vi "BRig_RT_panel_ExpStruct_v1,10.vi"(7 "input_setValues":bool, 11 "input_dataExp":u16[](array[numeric])) -> (3 "output_dataExp":u16[](array[numeric]))   [LabVIEW 2014]
panel:
  in  "I_Cue2":bool
  in  "T_Cue2_LED_max":u16=1000 caption="Max" min=5 max=5000 step=5
  in  "T_Cue2_LED_min":u16=1000 caption="Min" min=5 max=5000 step=5
  in  "T_Cue2_LED_step":u16=1000 caption="Penalty" min=1 max=10000 step=1
  in  "T_Cue2_Audio_max":u16=1000 caption="Max" min=5 max=5000 step=5
  in  "T_Cue2_Audio_min":u16=1000 caption="Min" min=5 max=5000 step=5
  in  "T_Cue2_Audio_step":u16=1000 caption="Penalty" min=1 max=10000 step=1
  in  "T_ENL2_step":u16=100 caption="Penalty" min=10 max=10000 step=10
  in  "T_ENL2_max":u16=1000 caption="Max" min=250 max=10000 step=250
  in  "T_ENL2_min":u16=1000 caption="Min" min=250 max=10000 step=250
  in  "ClosedLoop_LaserHold_l2":bool
  in  "ClosedLoop_LaserHold_l1":bool
  in  "FreeReward_Count2":u16
  in  "FreeReward_Count1":u16
  in  "FreeReward_Switch":bool
  in  "T_CuePenalty":u16=1000 caption="Penalty" min=1 max=10000 step=1
  in  "T_ENLPenalty":u16=100 caption="Penalty" min=10 max=10000 step=10
  in  "LaserSwitch_Probability_L1":u16
  in  "LaserSwitch":u16(slide) max=3 step=1 scale=0.0..3.0
  in  "I_allReward":bool caption="NonSpecific Lick Direction"
  in  "Tcycle_Reward_max_R":u16=1000 caption="Max" min=5 max=5000 step=5
  in  "Tcycle_Reward_min_R":u16=1000 caption="Min" min=5 max=5000 step=5
  in  "Tcycle_Reward_step_R":u16=1000 caption="Penalty" min=1 max=10000 step=1
  in  "Tcycle_Reward_max_L":u16=1000 caption="Max" min=5 max=5000 step=5
  in  "Tcycle_Reward_min_L":u16=1000 caption="Min" min=5 max=5000 step=5
  in  "Tcycle_Reward_step_L":u16=1000 caption="Penalty" min=1 max=10000 step=1
  in  "T_Cue_LED_max":u16=1000 caption="Max" min=5 max=5000 step=5
  in  "T_Cue_LED_min":u16=1000 caption="Min" min=5 max=5000 step=5
  in  "T_Cue_LED_step":u16=1000 caption="Penalty" min=1 max=10000 step=1
  in  "SolenoidProbability_L":u16=100 caption="Reward Time [ms]" min=1 max=1000 step=1
  in  "SolenoidProbability_R":u16=100 caption="Reward Time [ms]" min=1 max=1000 step=1
  in  "T_Cue_Audio_max":u16=1000 caption="Max" min=5 max=5000 step=5
  in  "T_Cue_Audio_min":u16=1000 caption="Min" min=5 max=5000 step=5
  in  "BUR_max":u16 caption="Count Reward Structure  (0 = off)"
  in  "Tcycle_Timeout":u16=1000 caption="Timeout Time [ms]" min=10 max=10000 step=1
  in  "Tcycle_Wrong":u16=1000 caption="Wrong Time [ms]" min=10 max=10000 step=1
  in  "Tcycle_Selection":u16=1000 caption="Answer Time [ms]" min=1 max=10000 step=1
  in  "Tcycle_RewardPost":u16=1000 caption="Consumption Time [ms]" min=250 max=10000 step=250
  in  "TpB_Max_R":u16=4 caption="Max TrialsPerBlock" min=1 max=12 step=1
  in  "TpB_Min_R":u16=4 caption="Min TrialsPerBlock" min=1 max=12 step=1
  in  "TpB_Max_L":u16=4 caption="Max TrialsPerBlock" min=1 max=12 step=1
  in  "TpB_Min_L":u16=4 caption="Min TrialsPerBlock" min=1 max=12 step=1
  in  "BUR_min":u16 caption="Count Reward Structure\n(0 = off)"
  in  "TrialUntilReward":bool caption="Ignore Wrong Selection"
  in  "T_Cue_Audio_step":u16=1000 caption="Penalty" min=1 max=10000 step=1
  in  "T_ENL_step":u16=100 caption="Penalty" min=10 max=10000 step=10
  in  "T_ENL_max":u16=1000 caption="Max" min=250 max=10000 step=250
  in  "T_ENL_min":u16=1000 caption="Min" min=250 max=10000 step=250
  # "Experiment Task Structure"
  # "Min            Max               Step        Penalty"
  # "(Laser1 or Laser2)\nLaser1 probability"
  # "Enforced\nNonLick"
  # "Cue Audio"
  # "(ClosedLoop Structure)"
  # "Hold Laser1"
  # "Hold Laser2"
  # "Cue LED"
  # "Min            Max               Step"
  # "ENL 2"
  # "Cue 2 Audio"
  # "Cue 2 LED"
  # "Selection"
  # "Min"
  # "Max"
  # "Reward - Dispense Water"
  # "Min            Max            StepSize"
  # "Left"
  # "Trial Per Block Structure \n               Left                        Right"
  # "Right"
  # "Min"
  # "Dispense Water Probability"
  # "Max"
  # "%"
  # "Left"
  # "Right"
  # "%"
  # "Give Reward\nIf Too Many Errors"
  # "Reward - Consumption"
  # "# consecutive ReBiasing trials"
  # "Penalty - Wrong Choice"
  # "# consecutive NonForcedError trials"
  # "Penalty - Choice Timeout"
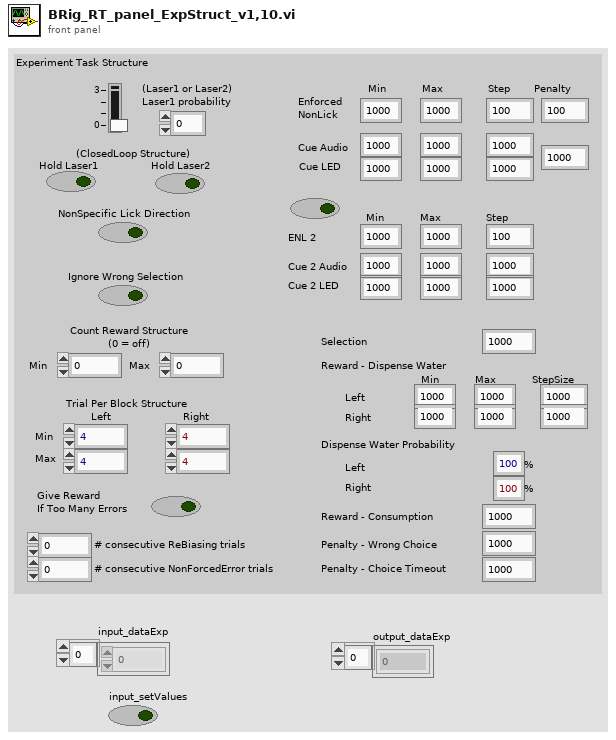
[diagram p1: front panel]
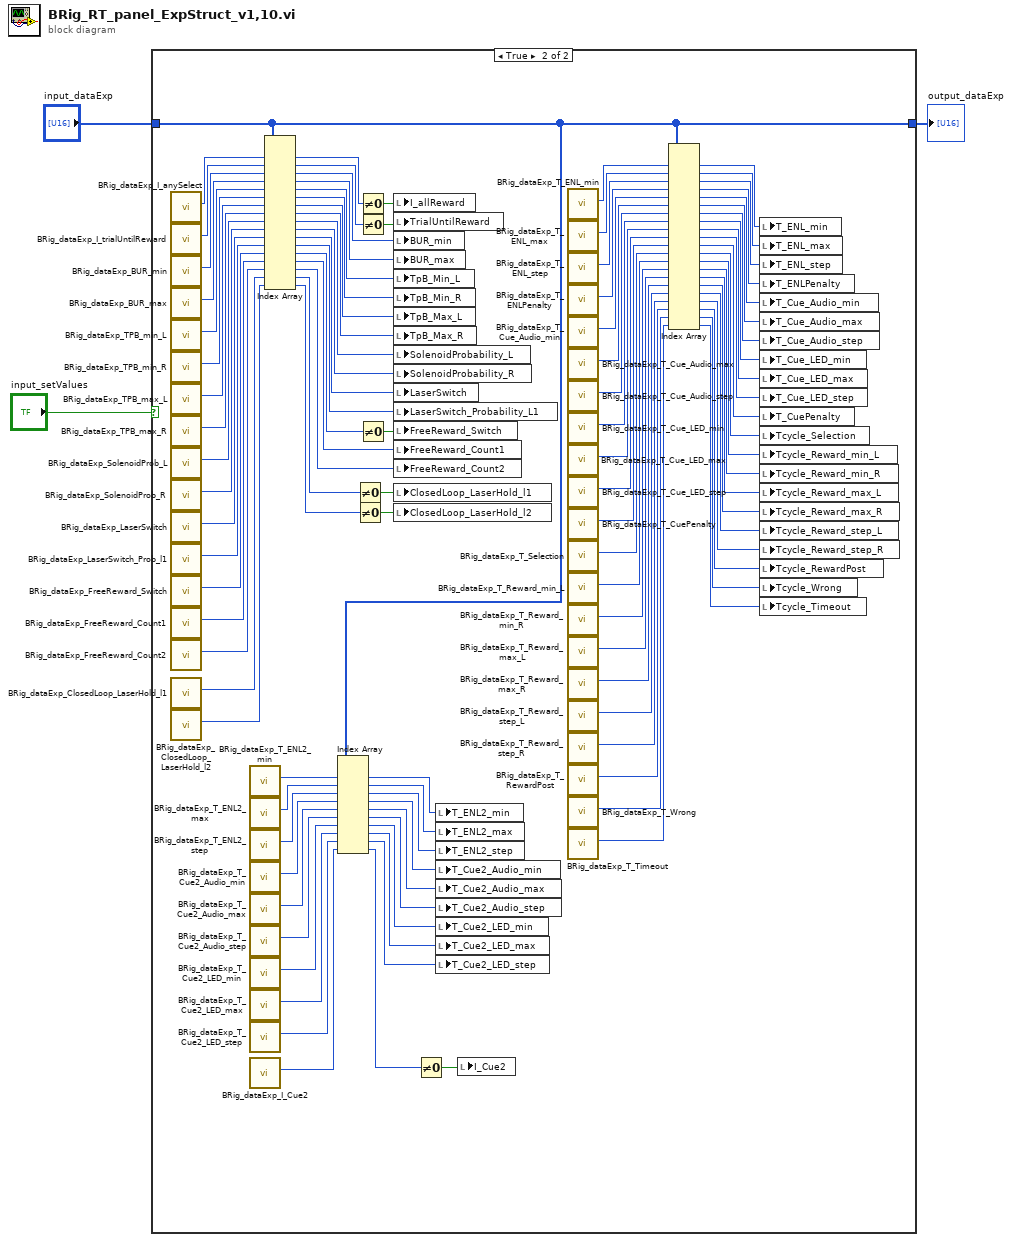
[diagram p0: block diagram]
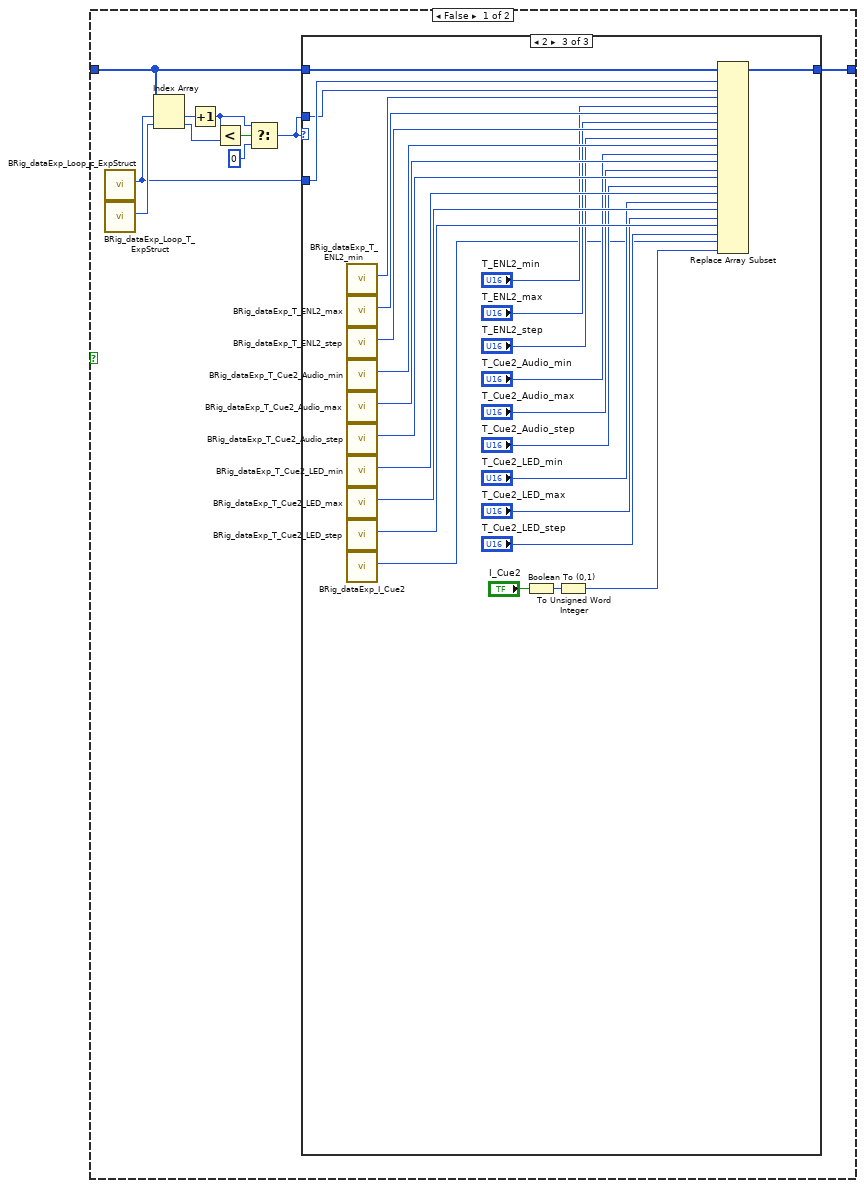
[diagram p2: hidden frame]
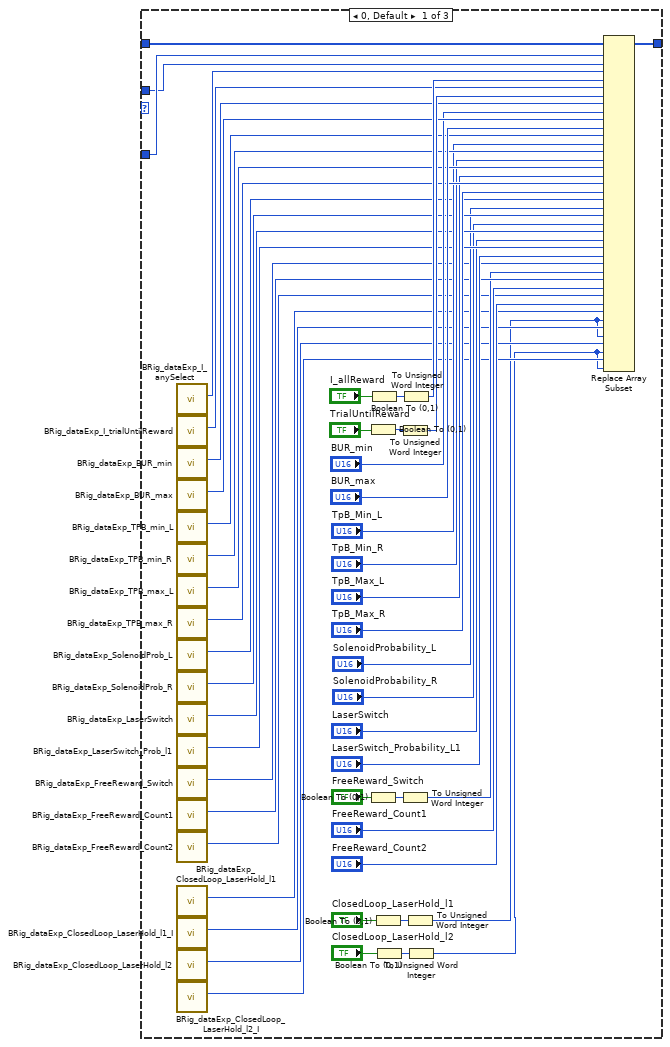
[diagram p3: hidden frame]
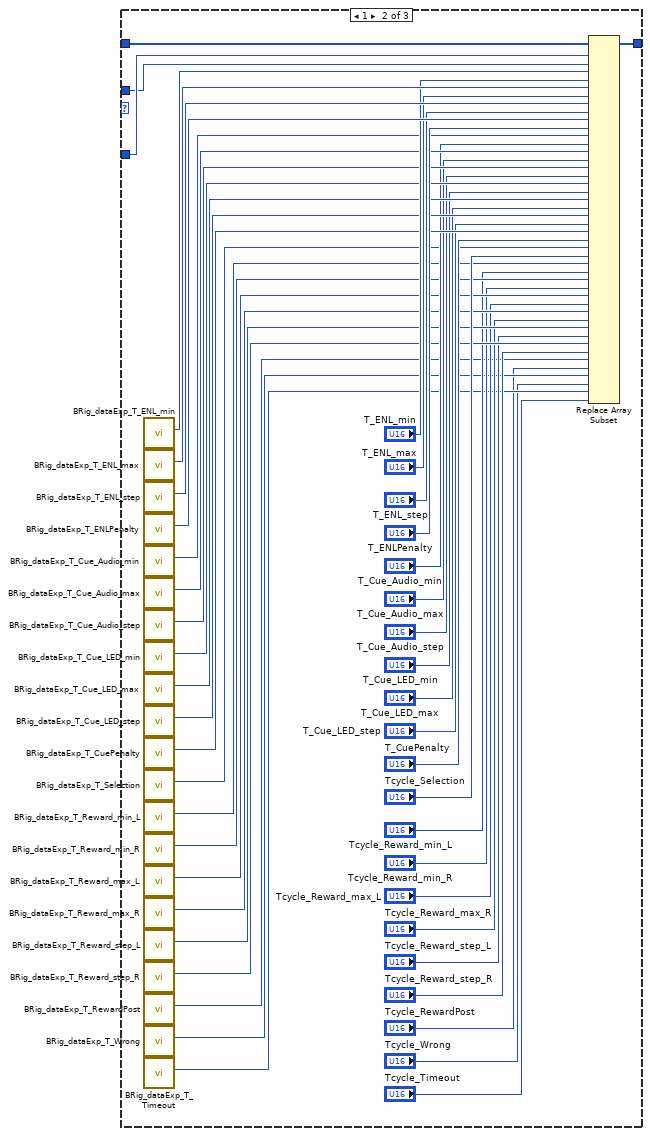
[diagram p4: hidden frame]
diagram:
  n1 = case shown="True" "input_setValues" {
    tunnel: [w13 w157] -> w3
    tunnel: "input_dataExp" -> [w12 w157]
    frame False {
      n2 = call "BRig_dataExp_Loop_c_ExpStruct.vi"() -> ("output_Loop_c_ExpStruct"=w6:i32)  [unwired: 11 in]
      n3 = call "BRig_dataExp_Loop_T_ExpStruct.vi"() -> ("output_Loop_T_ExpStruct"=w11:i32)  [unwired: 11 in]
      n4 = Index Array(array=w12, index #1=w6, index #2=w11) -> (element #1=w10:u16, element #2=w9:u16)
      n5 = Increment(x=w10) -> (x+1=w5:u16)
      n6 = Less?(x=w5, y=w9) -> (x < y?=w8:bool)
      n7 = Select(t=w5, s=w8, f=u16 0) -> (s? t:f=w4:u16)
      n8 = case shown="2" w4 {
        tunnel: w12 -> [w63 w109 w135]
        tunnel: [w62 w108 w134] -> w13
        tunnel: w6 -> [w33 w107 w133]
        tunnel: w4 -> [w32 w106 w132]
        frame 0, Default {
          n9 = call "BRig_dataExp_I_anySelect.vi"() -> ("output_I_anySelect"=w61:i32)  [unwired: 11 in]
          n10 = call "BRig_dataExp_I_trialUntilReward.vi"() -> ("output_I_trialUntilReward"=w57:i32)  [unwired: 11 in]
          n11 = call "BRig_dataExp_BUR_min.vi"() -> ("output_BUR_min"=w53:i32)  [unwired: 11 in]
          n12 = call "BRig_dataExp_BUR_max.vi"() -> ("output_BUR_max"=w52:i32)  [unwired: 11 in]
          n13 = call "BRig_dataExp_TPB_min_L.vi"() -> ("output_TPB_min_L"=w49:i32)  [unwired: 11 in]
          n14 = call "BRig_dataExp_TPB_min_R.vi"() -> ("output_TPB_min_R"=w48:i32)  [unwired: 11 in]
          n15 = call "BRig_dataExp_TPB_max_L.vi"() -> ("output_TPB_max_L"=w47:i32)  [unwired: 11 in]
          n16 = call "BRig_dataExp_TPB_max_R.vi"() -> ("output_TPB_max_R"=w46:i32)  [unwired: 11 in]
          n17 = call "BRig_dataExp_SolenoidProb_L.vi"() -> ("output_SolenoidProbability_L"=w41:i32)  [unwired: 11 in]
          n18 = call "BRig_dataExp_SolenoidProb_R.vi"() -> ("output_SolenoidProbability_R"=w40:i32)  [unwired: 11 in]
          n19 = call "BRig_dataExp_LaserSwitch.vi"() -> ("output_LaserSwitch"=w39:i32)  [unwired: 11 in]
          n20 = call "BRig_dataExp_LaserSwitch_Prob_l1.vi"() -> ("output_LaserSwitch_Probability_L1"=w38:i32)  [unwired: 11 in]
          n21 = call "BRig_dataExp_FreeReward_Switch.vi"() -> ("output_FreeReward_Switch"=w29:i32)  [unwired: 11 in]
          n22 = call "BRig_dataExp_FreeReward_Count1.vi"() -> ("output_FreeReward_Count"=w28:i32)  [unwired: 11 in]
          n23 = call "BRig_dataExp_FreeReward_Count2.vi"() -> ("output_FreeReward_Count"=w25:i32)  [unwired: 11 in]
          n24 = call "BRig_dataExp_ClosedLoop_LaserHold_l1.vi"() -> ("output_CloseLoop_LaserHold_l1"=w23:i32)  [unwired: 11 in]
          n25 = call "BRig_dataExp_ClosedLoop_LaserHold_l1_I.vi"() -> ("output_CloseLoop_LaserHold_l1_I"=w22:i32)  [unwired: 11 in]
          n26 = call "BRig_dataExp_ClosedLoop_LaserHold_l2.vi"() -> ("output_CloseLoop_LaserHold_l2"=w21:i32)  [unwired: 11 in]
          n27 = call "BRig_dataExp_ClosedLoop_LaserHold_l2_I.vi"() -> ("output_CloseLoop_LaserHold_l2_I"=w20:i32)  [unwired: 11 in]
          n28 = Boolean To (0,1)(Boolean="TrialUntilReward") -> (0, 1=w56:i16)
          n29 = Boolean To (0,1)(Boolean="FreeReward_Switch") -> (0, 1=w31:i16)
          n30 = Boolean To (0,1)(Boolean="I_allReward") -> (0, 1=w59:i16)
          n31 = Boolean To (0,1)(Boolean="ClosedLoop_LaserHold_l1") -> (0, 1=w19:i16)
          n32 = Boolean To (0,1)(Boolean="ClosedLoop_LaserHold_l2") -> (0, 1=w17:i16)
          n33 = To Unsigned Word Integer(number=w56) -> (unsigned 16bit integer=w54:u16)
          n34 = To Unsigned Word Integer(number=w31) -> (unsigned 16bit integer=w27:u16)
          n35 = To Unsigned Word Integer(number=w59) -> (unsigned 16bit integer=w58:u16)
          n36 = To Unsigned Word Integer(number=w19) -> (unsigned 16bit integer=w15:u16)
          n37 = To Unsigned Word Integer(number=w17) -> (unsigned 16bit integer=w14:u16)
          n38 = Replace Array Subset(array=w63, new element #1=w32, index #1=w33, new element #2=w58, index #2=w61, new element #3=w54, index #3=w57, new element #4="BUR_min", index #4=w53, new element #5="BUR_max", index #5=w52, new element #6="TpB_Min_L", index #6=w49, new element #7="TpB_Min_R", index #7=w48, new element #8="TpB_Max_L", index #8=w47, new element #9="TpB_Max_R", index #9=w46, new element #10="SolenoidProbability_L", index #10=w41, new element #11="SolenoidProbability_R", index #11=w40, new element #12="LaserSwitch", index #12=w39, new element #13="LaserSwitch_Probability_L1", index #13=w38, new element #14=w27, index #14=w29, new element #15="FreeReward_Count1", index #15=w28, new element #16="FreeReward_Count2", index #16=w25, new element #17=w15, index #17=w23, new element #18=w15, index #18=w22, new element #19=w14, index #19=w21, new element #20=w14, index #20=w20) -> (w62:u16[])
        }
        frame 1 {
          n39 = call "BRig_dataExp_T_ENL_min.vi"() -> ("output_T_ENL_min"=w105:i32)  [unwired: 11 in]
          n40 = call "BRig_dataExp_T_ENL_max.vi"() -> ("output_T_ENL_max"=w104:i32)  [unwired: 11 in]
          n41 = call "BRig_dataExp_T_ENL_step.vi"() -> ("output_T_ENL_step"=w103:i32)  [unwired: 11 in]
          n42 = call "BRig_dataExp_T_ENLPenalty.vi"() -> ("output_ENL_penalty"=w102:i32)  [unwired: 11 in]
          n43 = call "BRig_dataExp_T_Cue_Audio_min.vi"() -> ("output_T_Cue_Audio_min"=w97:i32)  [unwired: 11 in]
          n44 = call "BRig_dataExp_T_Cue_Audio_max.vi"() -> ("output_T_Cue_Audio_max"=w96:i32)  [unwired: 11 in]
          n45 = call "BRig_dataExp_T_Cue_Audio_step.vi"() -> ("output_T_Cue_Audio_step"=w95:i32)  [unwired: 11 in]
          n46 = call "BRig_dataExp_T_Cue_LED_min.vi"() -> ("output_T_Cue_LED_min"=w94:i32)  [unwired: 11 in]
          n47 = call "BRig_dataExp_T_Cue_LED_max.vi"() -> ("output_T_Cue_LED_max"=w93:i32)  [unwired: 11 in]
          n48 = call "BRig_dataExp_T_Cue_LED_step.vi"() -> ("output_T_Cue_LED_step"=w92:i32)  [unwired: 11 in]
          n49 = call "BRig_dataExp_T_CuePenalty.vi"() -> ("output_T_CuePenalty"=w91:i32)  [unwired: 11 in]
          n50 = call "BRig_dataExp_T_Selection.vi"() -> ("output_T_Selection"=w83:i32)  [unwired: 11 in]
          n51 = call "BRig_dataExp_T_Reward_min_L.vi"() -> ("output_Tcycle_Reward_min_L"=w81:i32)  [unwired: 11 in]
          n52 = call "BRig_dataExp_T_Reward_min_R.vi"() -> ("output_T_Reward_min_R"=w80:i32)  [unwired: 11 in]
          n53 = call "BRig_dataExp_T_Reward_max_L.vi"() -> ("output_T_Reward_max_L"=w79:i32)  [unwired: 11 in]
          n54 = call "BRig_dataExp_T_Reward_max_R.vi"() -> ("output_T_Reward_max_R"=w78:i32)  [unwired: 11 in]
          n55 = call "BRig_dataExp_T_Reward_step_L.vi"() -> ("output_T_Reward_step_L"=w77:i32)  [unwired: 11 in]
          n56 = call "BRig_dataExp_T_Reward_step_R.vi"() -> ("output_T_Reward_step_R"=w76:i32)  [unwired: 11 in]
          n57 = call "BRig_dataExp_T_RewardPost.vi"() -> ("output_T_RewardPost"=w69:i32)  [unwired: 11 in]
          n58 = call "BRig_dataExp_T_Wrong.vi"() -> ("output_T_Wrong"=w68:i32)  [unwired: 11 in]
          n59 = call "BRig_dataExp_T_Timeout.vi"() -> ("output_T_Timeout"=w67:i32)  [unwired: 11 in]
          n60 = Replace Array Subset(array=w109, new element #1=w106, index #1=w107, new element #2="T_ENL_min", index #2=w105, new element #3="T_ENL_max", index #3=w104, new element #4="T_ENL_step", index #4=w103, new element #5="T_ENLPenalty", index #5=w102, new element #6="T_Cue_Audio_min", index #6=w97, new element #7="T_Cue_Audio_max", index #7=w96, new element #8="T_Cue_Audio_step", index #8=w95, new element #9="T_Cue_LED_min", index #9=w94, new element #10="T_Cue_LED_max", index #10=w93, new element #11="T_Cue_LED_step", index #11=w92, new element #12="T_CuePenalty", index #12=w91, new element #13="Tcycle_Selection", index #13=w83, new element #14="Tcycle_Reward_min_L", index #14=w81, new element #15="Tcycle_Reward_min_R", index #15=w80, new element #16="Tcycle_Reward_max_L", index #16=w79, new element #17="Tcycle_Reward_max_R", index #17=w78, new element #18="Tcycle_Reward_step_L", index #18=w77, new element #19="Tcycle_Reward_step_R", index #19=w76, new element #20="Tcycle_RewardPost", index #20=w69, new element #21="Tcycle_Wrong", index #21=w68, new element #22="Tcycle_Timeout", index #22=w67) -> (w108:u16[])
        }
        frame 2 {
          n61 = call "BRig_dataExp_T_ENL2_min.vi"() -> ("output_T_ENL2_min"=w131:i32)  [unwired: 11 in]
          n62 = call "BRig_dataExp_T_ENL2_max.vi"() -> ("output_T_ENL2_max"=w130:i32)  [unwired: 11 in]
          n63 = call "BRig_dataExp_T_ENL2_step.vi"() -> ("output_T_ENL2_step"=w129:i32)  [unwired: 11 in]
          n64 = call "BRig_dataExp_T_Cue2_Audio_min.vi"() -> ("output_T_Cue2_Audio_min"=w128:i32)  [unwired: 11 in]
          n65 = call "BRig_dataExp_T_Cue2_Audio_max.vi"() -> ("output_T_Cue2_Audio_max"=w127:i32)  [unwired: 11 in]
          n66 = call "BRig_dataExp_T_Cue2_Audio_step.vi"() -> ("output_T_Cue2_Audio_step"=w126:i32)  [unwired: 11 in]
          n67 = call "BRig_dataExp_T_Cue2_LED_min.vi"() -> ("output_T_Cue2_LED_min"=w125:i32)  [unwired: 11 in]
          n68 = call "BRig_dataExp_T_Cue2_LED_max.vi"() -> ("output_T_Cue2_LED_max"=w124:i32)  [unwired: 11 in]
          n69 = call "BRig_dataExp_T_Cue2_LED_step.vi"() -> ("output_T_Cue2_LED_step"=w123:i32)  [unwired: 11 in]
          n70 = call "BRig_dataExp_I_Cue2.vi"() -> ("output_I_Cue2"=w113:i32)  [unwired: 11 in]
          n71 = Boolean To (0,1)(Boolean="I_Cue2") -> (0, 1=w111:i16)
          n72 = To Unsigned Word Integer(number=w111) -> (unsigned 16bit integer=w110:u16)
          n73 = Replace Array Subset(array=w135, new element #1=w132, index #1=w133, new element #2="T_ENL2_min", index #2=w131, new element #3="T_ENL2_max", index #3=w130, new element #4="T_ENL2_step", index #4=w129, new element #5="T_Cue2_Audio_min", index #5=w128, new element #6="T_Cue2_Audio_max", index #6=w127, new element #7="T_Cue2_Audio_step", index #7=w126, new element #8="T_Cue2_LED_min", index #8=w125, new element #9="T_Cue2_LED_max", index #9=w124, new element #10="T_Cue2_LED_step", index #10=w123, new element #11=w110, index #11=w113) -> (w134:u16[])
        }
      }
    }
    frame True {
      n74 = call "BRig_dataExp_I_anySelect.vi"() -> ("output_I_anySelect"=w238:i32)  [unwired: 11 in]
      n75 = call "BRig_dataExp_I_trialUntilReward.vi"() -> ("output_I_trialUntilReward"=w237:i32)  [unwired: 11 in]
      n76 = call "BRig_dataExp_BUR_min.vi"() -> ("output_BUR_min"=w236:i32)  [unwired: 11 in]
      n77 = call "BRig_dataExp_BUR_max.vi"() -> ("output_BUR_max"=w235:i32)  [unwired: 11 in]
      n78 = call "BRig_dataExp_TPB_min_L.vi"() -> ("output_TPB_min_L"=w234:i32)  [unwired: 11 in]
      n79 = call "BRig_dataExp_TPB_min_R.vi"() -> ("output_TPB_min_R"=w233:i32)  [unwired: 11 in]
      n80 = call "BRig_dataExp_TPB_max_L.vi"() -> ("output_TPB_max_L"=w232:i32)  [unwired: 11 in]
      n81 = call "BRig_dataExp_TPB_max_R.vi"() -> ("output_TPB_max_R"=w231:i32)  [unwired: 11 in]
      n82 = call "BRig_dataExp_SolenoidProb_L.vi"() -> ("output_SolenoidProbability_L"=w230:i32)  [unwired: 11 in]
      n83 = call "BRig_dataExp_SolenoidProb_R.vi"() -> ("output_SolenoidProbability_R"=w229:i32)  [unwired: 11 in]
      n84 = call "BRig_dataExp_LaserSwitch.vi"() -> ("output_LaserSwitch"=w228:i32)  [unwired: 11 in]
      n85 = call "BRig_dataExp_LaserSwitch_Prob_l1.vi"() -> ("output_LaserSwitch_Probability_L1"=w227:i32)  [unwired: 11 in]
      n86 = call "BRig_dataExp_FreeReward_Switch.vi"() -> ("output_FreeReward_Switch"=w226:i32)  [unwired: 11 in]
      n87 = call "BRig_dataExp_FreeReward_Count1.vi"() -> ("output_FreeReward_Count"=w225:i32)  [unwired: 11 in]
      n88 = call "BRig_dataExp_FreeReward_Count2.vi"() -> ("output_FreeReward_Count"=w165:i32)  [unwired: 11 in]
      n89 = call "BRig_dataExp_ClosedLoop_LaserHold_l1.vi"() -> ("output_CloseLoop_LaserHold_l1"=w163:i32)  [unwired: 11 in]
      n90 = call "BRig_dataExp_ClosedLoop_LaserHold_l2.vi"() -> ("output_CloseLoop_LaserHold_l2"=w162:i32)  [unwired: 11 in]
      n91 = call "BRig_dataExp_T_ENL2_min.vi"() -> ("output_T_ENL2_min"=w156:i32)  [unwired: 11 in]
      n92 = call "BRig_dataExp_T_ENL2_max.vi"() -> ("output_T_ENL2_max"=w155:i32)  [unwired: 11 in]
      n93 = call "BRig_dataExp_T_ENL2_step.vi"() -> ("output_T_ENL2_step"=w154:i32)  [unwired: 11 in]
      n94 = call "BRig_dataExp_T_Cue2_Audio_min.vi"() -> ("output_T_Cue2_Audio_min"=w153:i32)  [unwired: 11 in]
      n95 = call "BRig_dataExp_T_Cue2_Audio_max.vi"() -> ("output_T_Cue2_Audio_max"=w152:i32)  [unwired: 11 in]
      n96 = call "BRig_dataExp_T_Cue2_Audio_step.vi"() -> ("output_T_Cue2_Audio_step"=w151:i32)  [unwired: 11 in]
      n97 = call "BRig_dataExp_T_Cue2_LED_min.vi"() -> ("output_T_Cue2_LED_min"=w150:i32)  [unwired: 11 in]
      n98 = call "BRig_dataExp_T_Cue2_LED_max.vi"() -> ("output_T_Cue2_LED_max"=w149:i32)  [unwired: 11 in]
      n99 = call "BRig_dataExp_T_Cue2_LED_step.vi"() -> ("output_T_Cue2_LED_step"=w148:i32)  [unwired: 11 in]
      n100 = call "BRig_dataExp_I_Cue2.vi"() -> ("output_I_Cue2"=w138:i32)  [unwired: 11 in]
      n101 = Index Array(array=w157, index #1=w238, index #2=w237, index #3=w236, index #4=w235, index #5=w234, index #6=w233, index #7=w232, index #8=w231, index #9=w230, index #10=w229, index #11=w228, index #12=w227, index #13=w226, index #14=w225, index #15=w165, index #16=w163, index #17=w162) -> (element #1=w221:u16, element #2=w220:u16, element #3=w219:u16, element #4=w218:u16, element #5=w217:u16, element #6=w216:u16, element #7=w215:u16, element #8=w214:u16, element #9=w213:u16, element #10=w212:u16, element #11=w211:u16, element #12=w210:u16, element #13=w209:u16, element #14=w208:u16, element #15=w164:u16, element #16=w159:u16, element #17=w158:u16)
      n102 = Index Array(array=w157, index #1=w156, index #2=w155, index #3=w154, index #4=w153, index #5=w152, index #6=w151, index #7=w150, index #8=w149, index #9=w148, index #10=w138) -> (element #1=w147:u16, element #2=w146:u16, element #3=w145:u16, element #4=w144:u16, element #5=w143:u16, element #6=w142:u16, element #7=w141:u16, element #8=w140:u16, element #9=w139:u16, element #10=w136:u16)
      n103 = Not Equal To 0?(x=w159) -> (x != 0?=w161:bool)
      n104 = Not Equal To 0?(x=w158) -> (x != 0?=w160:bool)
      n105 = Not Equal To 0?(x=w221) -> (x != 0?=w224:bool)
      n106 = Not Equal To 0?(x=w220) -> (x != 0?=w223:bool)
      n107 = Not Equal To 0?(x=w209) -> (x != 0?=w222:bool)
      n108 = local write "I_allReward"(w224) -> ()
      n109 = local write "TrialUntilReward"(w223) -> ()
      n110 = local write "BUR_min"(w219) -> ()
      n111 = local write "BUR_max"(w218) -> ()
      n112 = local write "TpB_Min_L"(w217) -> ()
      n113 = local write "TpB_Min_R"(w216) -> ()
      n114 = local write "TpB_Max_L"(w215) -> ()
      n115 = local write "TpB_Max_R"(w214) -> ()
      n116 = local write "SolenoidProbability_L"(w213) -> ()
      n117 = local write "SolenoidProbability_R"(w212) -> ()
      n118 = local write "LaserSwitch"(w211) -> ()
      n119 = local write "LaserSwitch_Probability_L1"(w210) -> ()
      n120 = local write "FreeReward_Switch"(w222) -> ()
      n121 = local write "FreeReward_Count1"(w208) -> ()
      n122 = local write "FreeReward_Count2"(w164) -> ()
      n123 = local write "ClosedLoop_LaserHold_l1"(w161) -> ()
      n124 = local write "ClosedLoop_LaserHold_l2"(w160) -> ()
      n125 = Not Equal To 0?(x=w136) -> (x != 0?=w137:bool)
      n126 = local write "T_ENL2_min"(w147) -> ()
      n127 = local write "T_ENL2_max"(w146) -> ()
      n128 = local write "T_ENL2_step"(w145) -> ()
      n129 = local write "T_Cue2_Audio_min"(w144) -> ()
      n130 = local write "T_Cue2_Audio_max"(w143) -> ()
      n131 = local write "T_Cue2_Audio_step"(w142) -> ()
      n132 = local write "T_Cue2_LED_min"(w141) -> ()
      n133 = local write "T_Cue2_LED_max"(w140) -> ()
      n134 = local write "T_Cue2_LED_step"(w139) -> ()
      n135 = local write "I_Cue2"(w137) -> ()
      n136 = call "BRig_dataExp_T_ENL_min.vi"() -> ("output_T_ENL_min"=w207:i32)  [unwired: 11 in]
      n137 = call "BRig_dataExp_T_ENL_max.vi"() -> ("output_T_ENL_max"=w206:i32)  [unwired: 11 in]
      n138 = call "BRig_dataExp_T_ENL_step.vi"() -> ("output_T_ENL_step"=w205:i32)  [unwired: 11 in]
      n139 = call "BRig_dataExp_T_ENLPenalty.vi"() -> ("output_ENL_penalty"=w204:i32)  [unwired: 11 in]
      n140 = call "BRig_dataExp_T_Cue_Audio_min.vi"() -> ("output_T_Cue_Audio_min"=w203:i32)  [unwired: 11 in]
      n141 = call "BRig_dataExp_T_Cue_Audio_max.vi"() -> ("output_T_Cue_Audio_max"=w202:i32)  [unwired: 11 in]
      n142 = call "BRig_dataExp_T_Cue_Audio_step.vi"() -> ("output_T_Cue_Audio_step"=w201:i32)  [unwired: 11 in]
      n143 = call "BRig_dataExp_T_Cue_LED_min.vi"() -> ("output_T_Cue_LED_min"=w200:i32)  [unwired: 11 in]
      n144 = call "BRig_dataExp_T_Cue_LED_max.vi"() -> ("output_T_Cue_LED_max"=w199:i32)  [unwired: 11 in]
      n145 = call "BRig_dataExp_T_Cue_LED_step.vi"() -> ("output_T_Cue_LED_step"=w198:i32)  [unwired: 11 in]
      n146 = call "BRig_dataExp_T_CuePenalty.vi"() -> ("output_T_CuePenalty"=w197:i32)  [unwired: 11 in]
      n147 = call "BRig_dataExp_T_Selection.vi"() -> ("output_T_Selection"=w196:i32)  [unwired: 11 in]
      n148 = call "BRig_dataExp_T_Reward_min_L.vi"() -> ("output_Tcycle_Reward_min_L"=w195:i32)  [unwired: 11 in]
      n149 = call "BRig_dataExp_T_Reward_min_R.vi"() -> ("output_T_Reward_min_R"=w194:i32)  [unwired: 11 in]
      n150 = call "BRig_dataExp_T_Reward_max_L.vi"() -> ("output_T_Reward_max_L"=w193:i32)  [unwired: 11 in]
      n151 = call "BRig_dataExp_T_Reward_max_R.vi"() -> ("output_T_Reward_max_R"=w192:i32)  [unwired: 11 in]
      n152 = call "BRig_dataExp_T_Reward_step_L.vi"() -> ("output_T_Reward_step_L"=w191:i32)  [unwired: 11 in]
      n153 = call "BRig_dataExp_T_Reward_step_R.vi"() -> ("output_T_Reward_step_R"=w190:i32)  [unwired: 11 in]
      n154 = call "BRig_dataExp_T_RewardPost.vi"() -> ("output_T_RewardPost"=w189:i32)  [unwired: 11 in]
      n155 = call "BRig_dataExp_T_Wrong.vi"() -> ("output_T_Wrong"=w188:i32)  [unwired: 11 in]
      n156 = call "BRig_dataExp_T_Timeout.vi"() -> ("output_T_Timeout"=w187:i32)  [unwired: 11 in]
      n157 = Index Array(array=w157, index #1=w207, index #2=w206, index #3=w205, index #4=w204, index #5=w203, index #6=w202, index #7=w201, index #8=w200, index #9=w199, index #10=w198, index #11=w197, index #12=w196, index #13=w195, index #14=w194, index #15=w193, index #16=w192, index #17=w191, index #18=w190, index #19=w189, index #20=w188, index #21=w187) -> (element #1=w186:u16, element #2=w185:u16, element #3=w184:u16, element #4=w183:u16, element #5=w182:u16, element #6=w181:u16, element #7=w180:u16, element #8=w179:u16, element #9=w178:u16, element #10=w177:u16, element #11=w176:u16, element #12=w175:u16, element #13=w174:u16, element #14=w173:u16, element #15=w172:u16, element #16=w171:u16, element #17=w170:u16, element #18=w169:u16, element #19=w168:u16, element #20=w167:u16, element #21=w166:u16)
      n158 = local write "T_ENL_min"(w186) -> ()
      n159 = local write "T_ENL_max"(w185) -> ()
      n160 = local write "T_ENL_step"(w184) -> ()
      n161 = local write "T_ENLPenalty"(w183) -> ()
      n162 = local write "T_Cue_Audio_min"(w182) -> ()
      n163 = local write "T_Cue_Audio_max"(w181) -> ()
      n164 = local write "T_Cue_Audio_step"(w180) -> ()
      n165 = local write "T_Cue_LED_min"(w179) -> ()
      n166 = local write "T_Cue_LED_max"(w178) -> ()
      n167 = local write "T_Cue_LED_step"(w177) -> ()
      n168 = local write "T_CuePenalty"(w176) -> ()
      n169 = local write "Tcycle_Selection"(w175) -> ()
      n170 = local write "Tcycle_Reward_min_L"(w174) -> ()
      n171 = local write "Tcycle_Reward_min_R"(w173) -> ()
      n172 = local write "Tcycle_Reward_max_L"(w172) -> ()
      n173 = local write "Tcycle_Reward_max_R"(w171) -> ()
      n174 = local write "Tcycle_Reward_step_L"(w170) -> ()
      n175 = local write "Tcycle_Reward_step_R"(w169) -> ()
      n176 = local write "Tcycle_RewardPost"(w168) -> ()
      n177 = local write "Tcycle_Wrong"(w167) -> ()
      n178 = local write "Tcycle_Timeout"(w166) -> ()
    }
  }
  "output_dataExp" <- w3
